vi "New Project.vi"(9 "DBSet":T1={"Server"="172.20.23.107", "DB"="HTPSDB", "PSW"="data'songyy", "User"="sa"}, 10 "UserID":string="L043460", 11 "厂区":string="清溪") -> ()   [LabVIEW 2011] (continued)
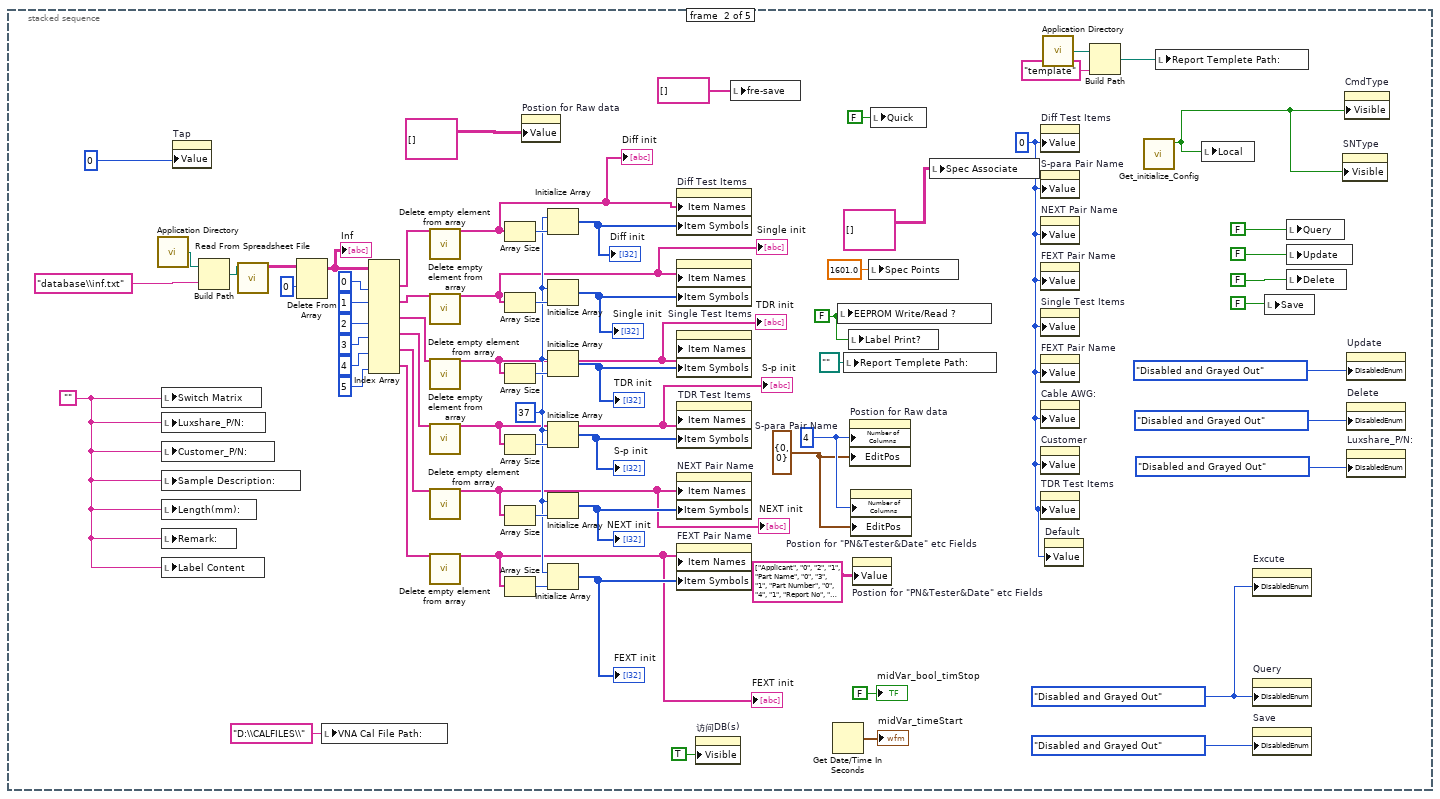
[diagram p5: hidden frame]
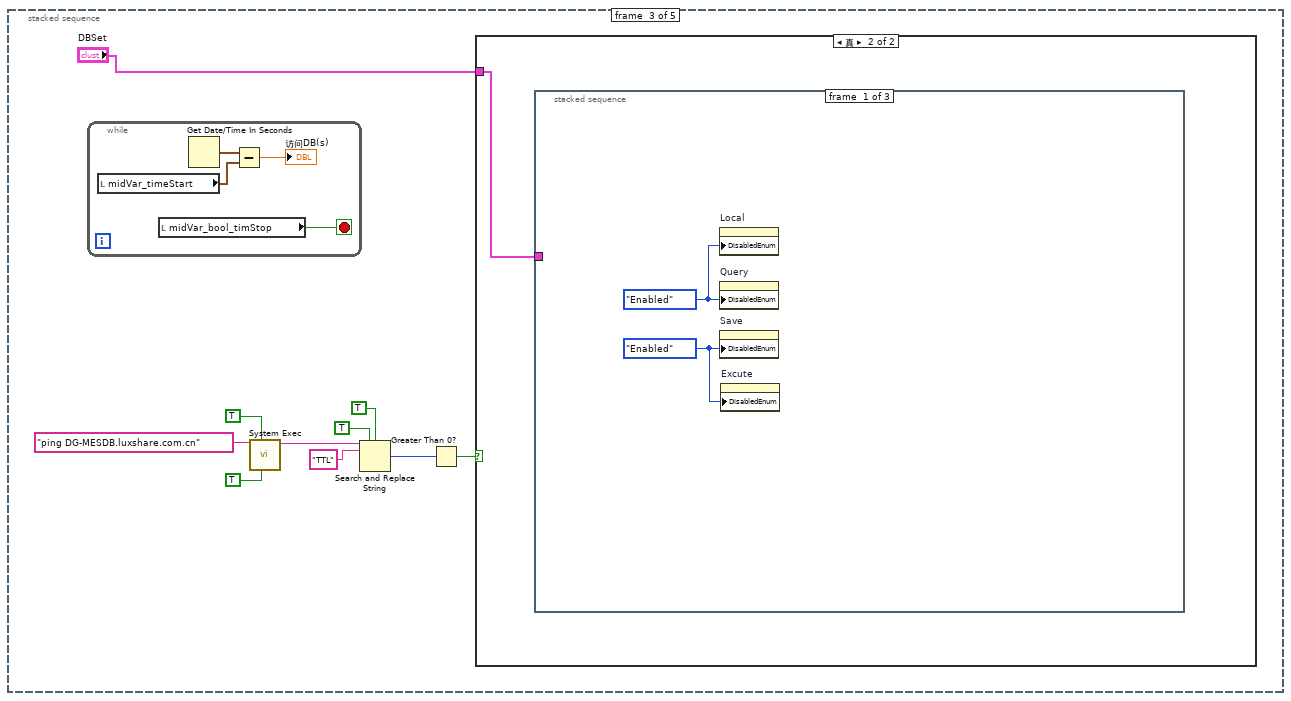
[diagram p6: hidden frame]
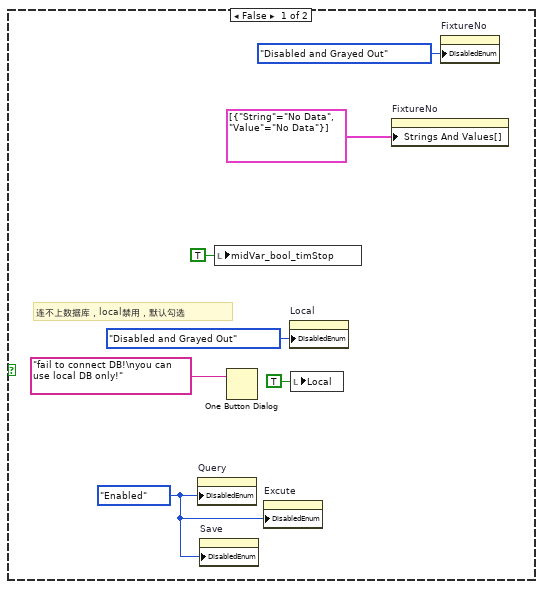
[diagram p7: hidden frame]
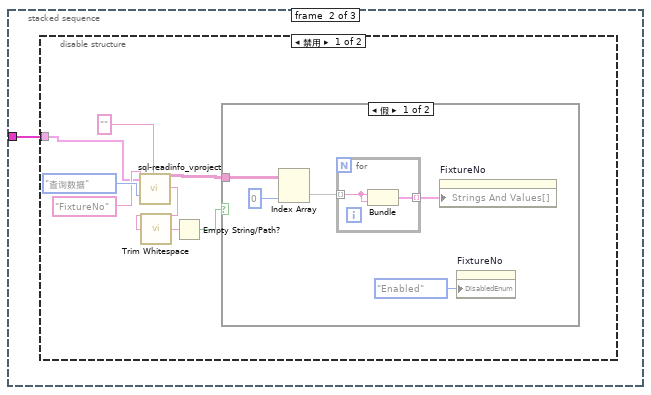
[diagram p8: hidden frame]
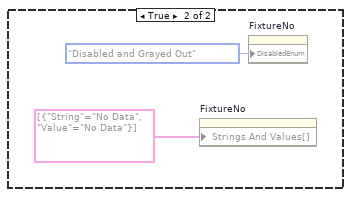
[diagram p9: hidden frame]
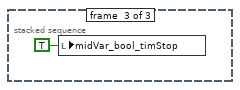
[diagram p11: hidden frame]
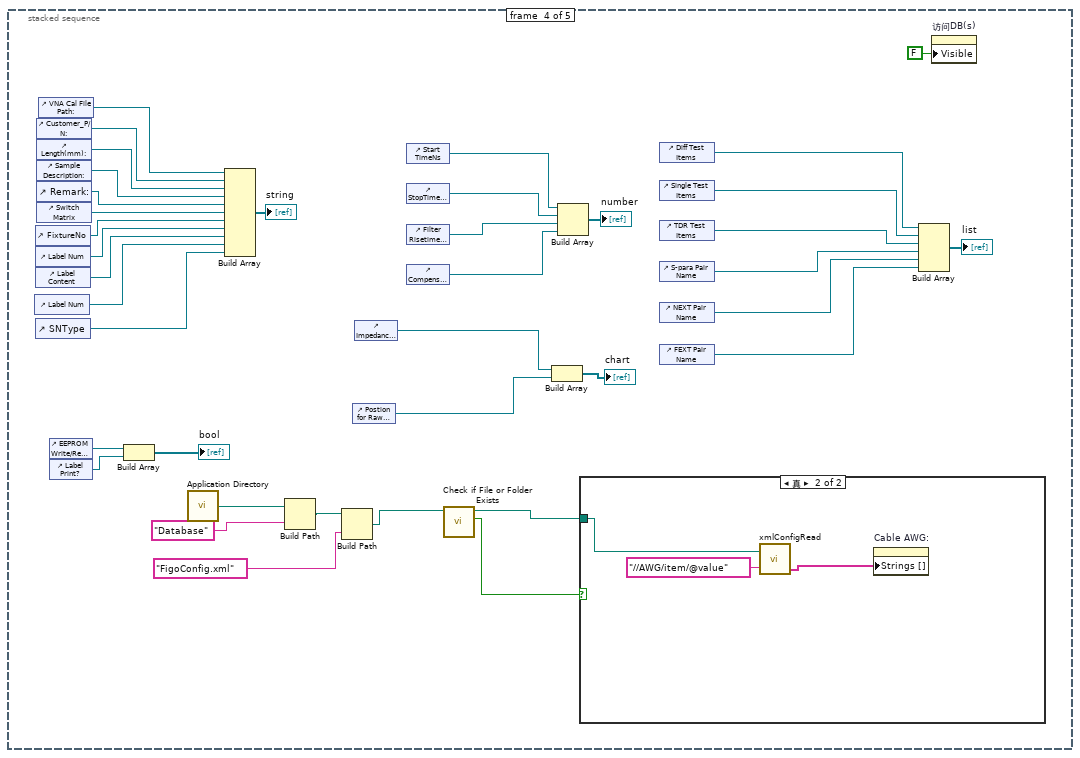
[diagram p12: hidden frame]
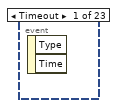
[diagram p14: hidden frame]
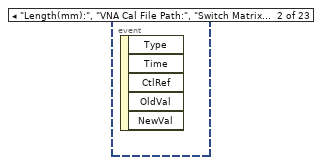
[diagram p15: hidden frame]
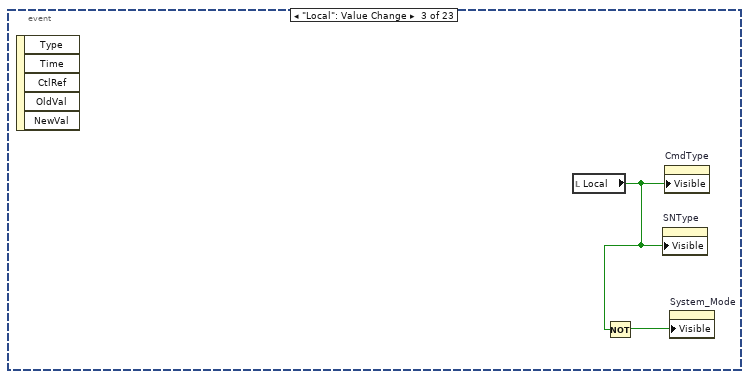
[diagram p16: hidden frame]
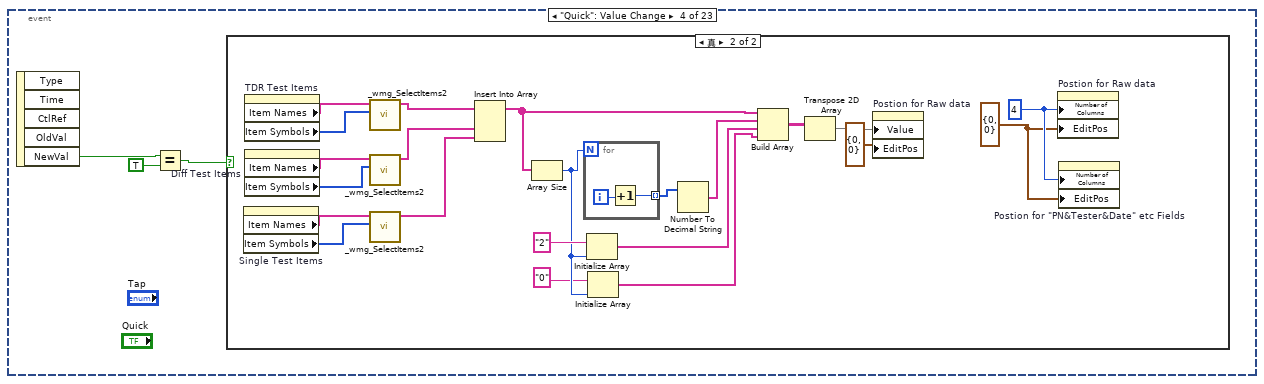
[diagram p17: hidden frame]
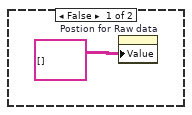
[diagram p18: hidden frame]
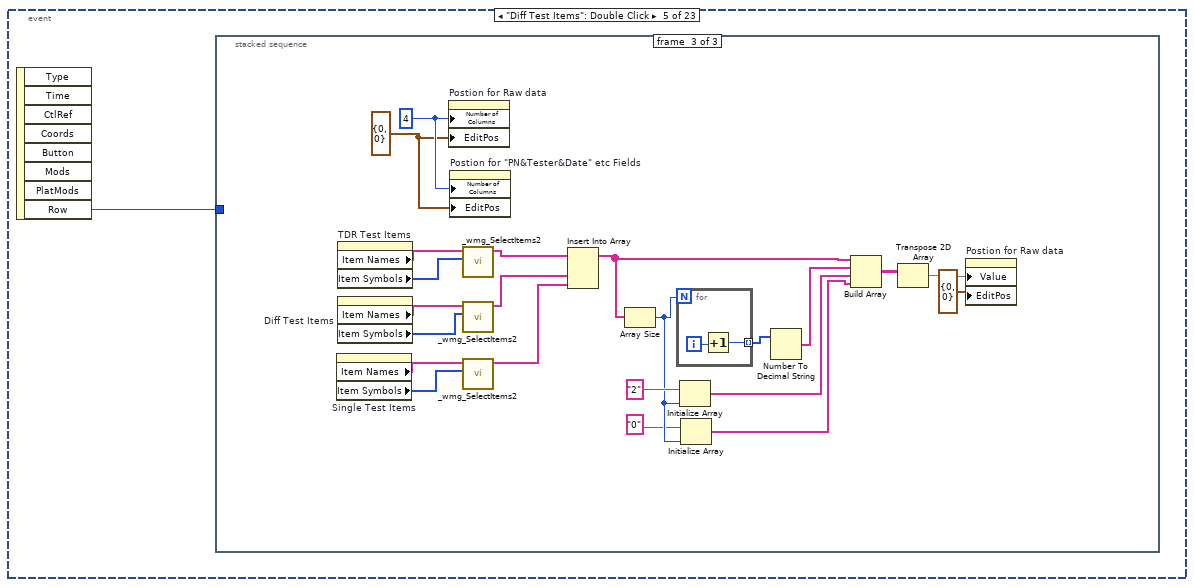
[diagram p19: hidden frame]
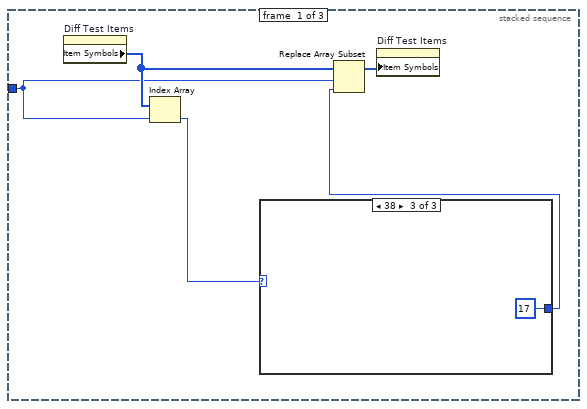
[diagram p20: hidden frame]
